vi "Delete Generated Server Code.vi"(8 "error in (no error)":errorcluster, 10 "Server Stub Name":string="Generated_server", 11 "Project Path":path) -> (0 "error out":errorcluster)   [LabVIEW 2019, in "gRPC Template Creation Utility.lvlib"]
uses:
  gRPC Template Creation Utility.lvlib
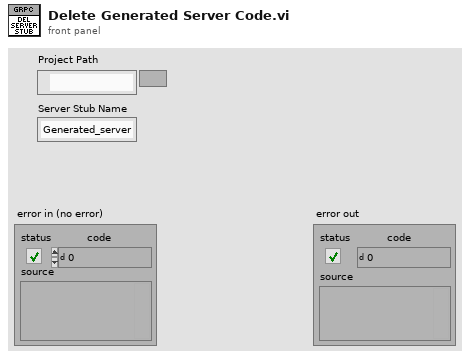
[diagram p1: front panel]
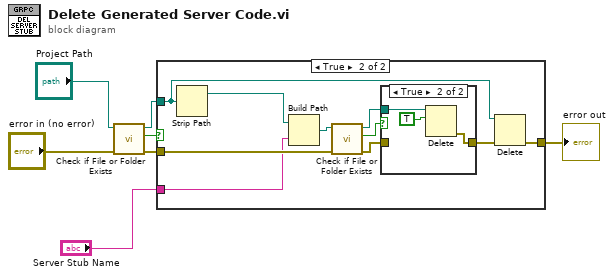
[diagram p0: block diagram]
diagram:
  n1 = call <vilib>:"Check if File or Folder Exists.vi"("error in (no error)"="error in (no error)", "path"="Project Path") -> ("error out"=w4:errorcluster, "file or folder exists?"=w6:bool, "dup path"=w5:path)  [unwired: 7 in]
  n2 = case shown="True" w6 {
    tunnel: w5 -> [_ w13]
    tunnel: w4 -> [w8 w11]
    tunnel: [w8 w10] -> w2
    tunnel: "Server Stub Name" -> [_ w9]
    frame False {
    }
    frame True {
      n3 = Strip Path(path=w13) -> (stripped path=w12:path)  [unwired: 1 out]
      n4 = Build Path(base path=w12, name or relative path=w9) -> (appended path=w18:path)
      n5 = call <vilib>:"Check if File or Folder Exists.vi"("error in (no error)"=w11, "path"=w18) -> ("error out"=w14:errorcluster, "file or folder exists?"=w16:bool, "dup path"=w17:path)  [unwired: 7 in]
      n6 = case shown="True" w16 {
        tunnel: w17 -> [_ w21]
        tunnel: [w19 w20] -> w15
        tunnel: w14 -> [w19 _]
        frame False {
        }
        frame True {
          n7 = Delete(path (use dialog)=w21, entire hierarchy (F)=TRUE) -> (error out=w20:errorcluster)  [unwired: 3 in, 2 out]
        }
      }
      n8 = Delete(path (use dialog)=w13, error in=w15) -> (error out=w10:errorcluster)  [unwired: 3 in, 2 out]
    }
  }
  "error out" <- w2
